vi "Facade.vi"(0 "Data In":T5, 2 "Display State In":T3={"X cursor"={"state"=enum."cursor and slider", "color"=0}, "Y cursor"={"state"=enum."cursor and slider", "color"=6618880}, "Scale Sliders"=FALSE}, 3 "Container State":T4) -> (6 "Data Out":T5, 7 "Display State Out":T3={"X cursor"={"state"=enum."cursor and slider", "color"=0}, "Y cursor"={"state"=enum."cursor and slider", "color"=6618880}, "Scale Sliders"=FALSE}, 8 "Action":T2)   [LabVIEW 2016, in "CursorImageControl.xctl"]
doc: "This is my documentation!!! Huzzahasdfasdf"
uses:
  CursorImageControl.xctl
  Data.ctl
  <vilib>/vision/Image Controls.llb/IMAQ Image.ctl
  <vilib>/_xctls/Container State.ctl
  State.ctl
  <vilib>/_xctls/Action.ctl
  <vilib>/Utility/miscctls.llb/LVPositionTypeDef.ctl
  PixelToMicron.vi
  <vilib>/_xctls/XControlSupport.lvlib
  <resource>/objmgr/IMAQImage.rc
panel:
  in  "X [mm]":dbl(slide) scale=-2.0..2.0 scale format="%#.2g"
  in  "Y [mm]":dbl(slide) scale=2.0..-2.0 scale format="%#.2g"
  out "Cursor Control":T1(plugin-control)
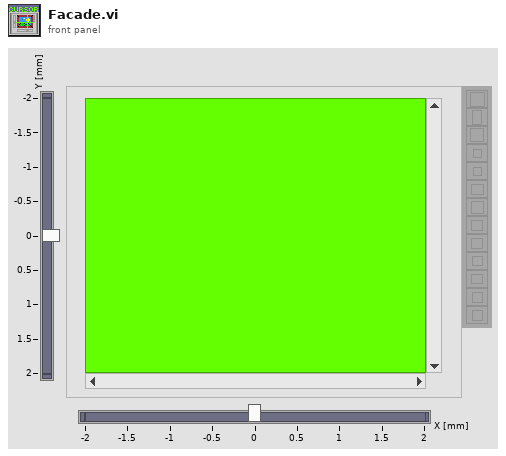
[diagram p1: front panel]
types:
  T1 = typedef "IMAQ Image.ctl" = refnum<image>
  T2 = typedef "XControlSupport.lvlib/Action.ctl" = cluster{"Data Changed?":bool, "State Changed?":bool, "Action Name":string}
  T3 = typedef "CursorImageControl.xctl/State.ctl" = cluster{"X cursor":cluster{"state":enum16{"cursor and slider", "cursor only", "hide all"}, "color":u32}, "Y cursor":cluster{"state":enum16{"cursor and slider", "cursor only", "hide all"}, "color":u32}, "Scale Sliders":bool}
  T4 = typedef "XControlSupport.lvlib/Container State.ctl" = cluster{"Indicator?":bool, "Run Mode?":bool, " Refnum":refnum<vi>}
  T5 = typedef "CursorImageControl.xctl/Data.ctl" = cluster{"Image":T1, "cursors":cluster{"X cursor":dbl, "Y cursor":dbl}}
  T6 = enum16{"cursor and slider", "cursor only", "hide all"}
  T7 = typedef "LVPositionTypeDef.ctl" = cluster{"Left":i32, "Top":i32}
  T8 = cluster{"state":enum16{"cursor and slider", "cursor only", "hide all"}, "state":enum16{"cursor and slider", "cursor only", "hide all"}}
  T9 = cluster{"Image":T1, cluster{"X [mm]":dbl, "Y [mm]":dbl}}
  T10 = typedef "LVBoundsTypeDef.ctl" = cluster{"Width":u32, "Height":u32}
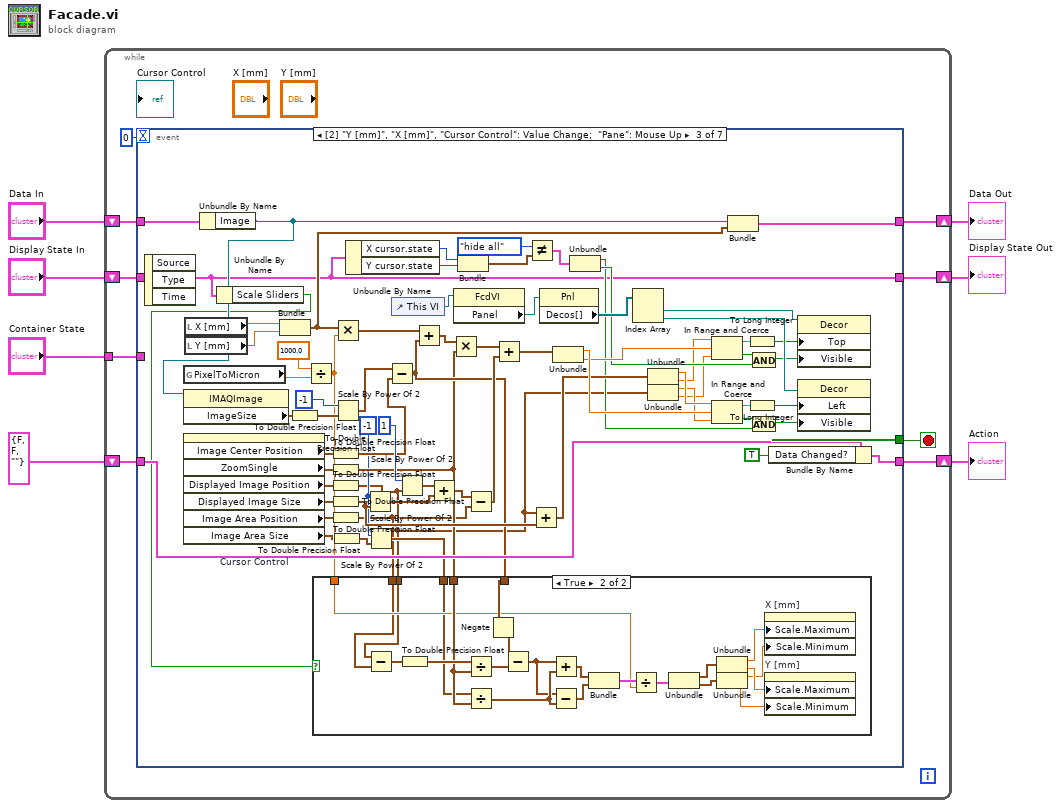
[diagram p0: block diagram]
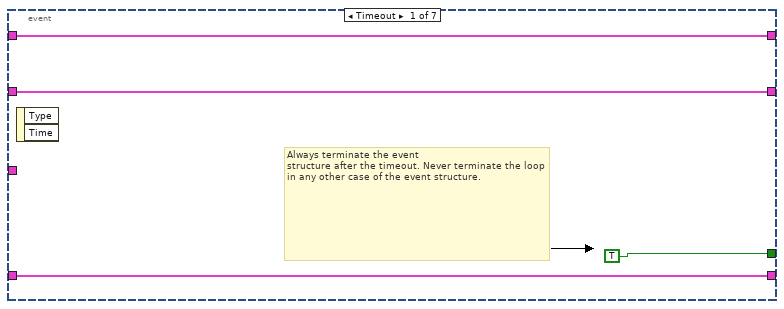
[diagram p2: hidden frame]
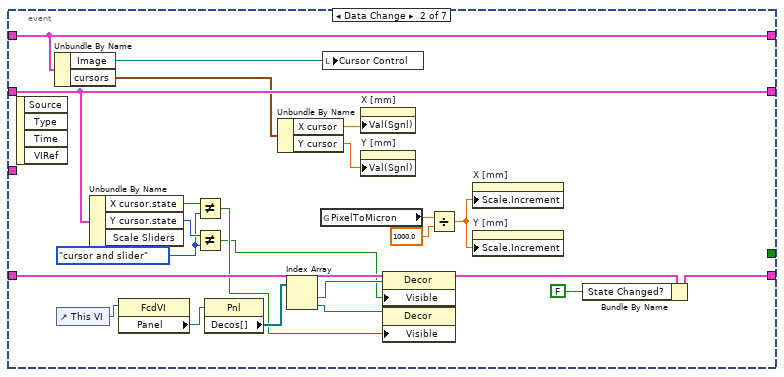
[diagram p3: hidden frame]
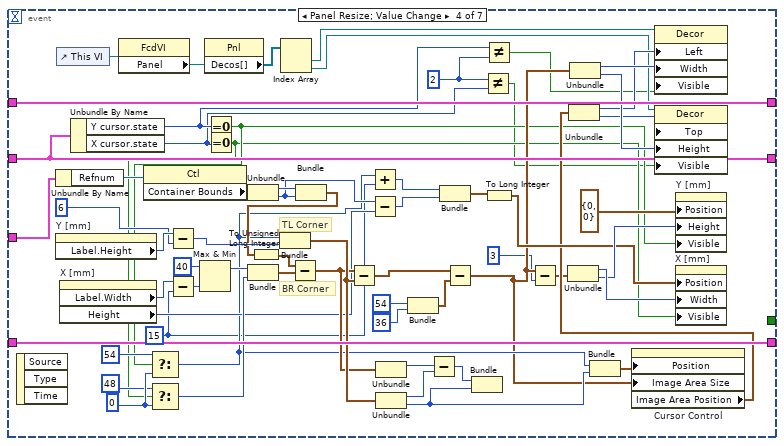
[diagram p5: hidden frame]
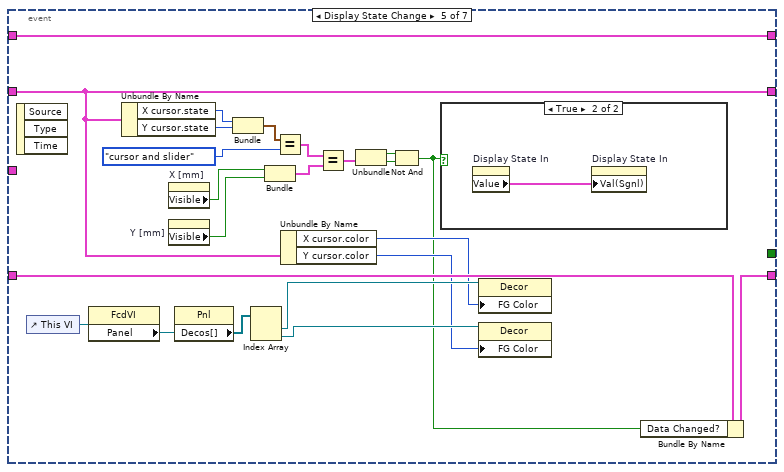
[diagram p6: hidden frame]
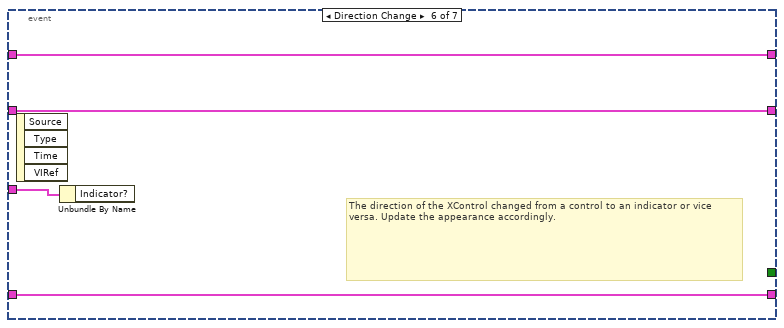
[diagram p8: hidden frame]
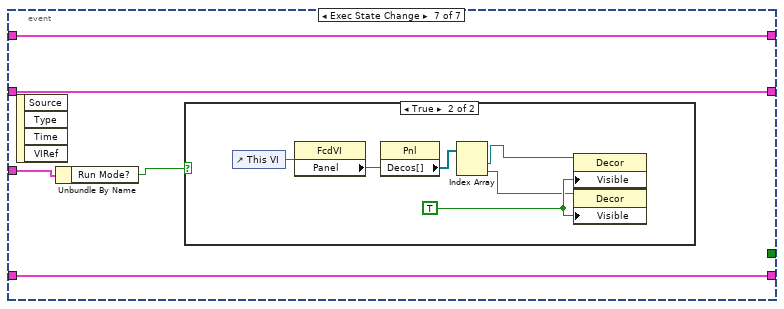
[diagram p9: hidden frame]
diagram:
  n1 = while {
    shift-right: [w15] -> w2
    shift-left: "Display State In" -> [w16]
    tunnel: "Container State" -> [w12]
    shift-right: [w8] -> w3
    shift-left: "Data In" -> [w9]
    shift-right: [w10] -> w1
    shift-left: T2 {"Data Changed?"=FALSE, "State Changed?"=FALSE, "Action Name"=""} ("Action") -> [w11]
    stop <- w14 stop-if-true
    n2 = event shown="[2] \"Y [mm]\", \"X [mm]\", \"Cursor Control\": Value Change;  \"Pane\": Mouse Up" {
      selector: _ -> [_ _ _ _ _ _ _]
      dyn-events: _ -> [_ _ _ _ _ _ _]
      timeout: 0 -> [_ _ _ _ _ _ _]
      tunnel: w16 -> [w18 w32 w56 w192 w201 w223 w226]
      tunnel: [w18 w32 w56 w192 w201 w223 w226] -> w15
      tunnel: [TRUE _ _ _ _ _ _] -> w14
      tunnel: w12 -> [_ _ _ w194 _ w224 w229]
      tunnel: w9 -> [w17 w39 w79 w196 w219 w221 w228]
      tunnel: [w17 w39 w62 w196 w219 w221 w228] -> w8
      tunnel: [w19 w41 w96 w195 w198 w222 w227] -> w10
      tunnel: w11 -> [w19 w42 w111 w195 w218 w222 w227]
      event Timeout {
        # "Always terminate the event\nstructure after the timeout. Never terminate the loop in any other case of the event structure."
        n3 = event-data() -> ()  [unwired: 1 in, 2 out]
      }
      event Data Change {
        w29 = T6."cursor and slider" ("X cursor.state")
        n4 = event-data() -> ()  [unwired: 1 in, 4 out]
        n5 = Unbundle By Name(w39) -> ("Image"=w26:T1, "cursors"=w21:cluster{"X cursor":dbl, "Y cursor":dbl})
        n6 = control-ref of="This VI"() -> (w34:refnum<vi>)
        n7 = Unbundle By Name(w32) -> ("X cursor.state"=w31:T6, "Y cursor.state"=w30:T6)  [unwired: 1 out]
        n8 = property class="FcdVI"(reference=w34) -> ("Panel"=w35:refnum<vi>)  [unwired: 1 in, 2 out]
        n9 = Not Equal?(x=w31, y=w29) -> (x != y?=w28:bool)
        n10 = Not Equal?(x=w30, y=w29) -> (x != y?=w27:bool)
        n11 = property class="Pnl"(reference=w35) -> ("Decos[]"=w36:refnum<vi>[])  [unwired: 1 in, 2 out]
        n12 = Unbundle By Name(w21) -> ("X cursor"=w22:dbl, "Y cursor"=w33:dbl)
        n13 = Index Array(array=w36) -> (element #1=w37:refnum<vi>, element #2=w38:refnum<vi>)  [unwired: 2 in]
        n14 = global read "PixelToMicron.vi" "PixelToMicron"() -> (w24:dbl)
        n15 = local write "Cursor Control"(w26) -> ()
        n16 = property on="X [mm]" class="Slide (strict)"("Val(Sgnl)"=w22) -> ()  [unwired: 2 in, 2 out]
        n17 = property on="Y [mm]" class="Slide (strict)"("Val(Sgnl)"=w33) -> ()  [unwired: 2 in, 2 out]
        n18 = property class="Decor"(reference=w37, "Visible"=w27) -> ()  [unwired: 1 in, 2 out]
        n19 = property class="Decor"(reference=w38, "Visible"=w28) -> ()  [unwired: 1 in, 2 out]
        n20 = Divide(x=w24, y=1000.0) -> (x/y=w23:dbl)
        n21 = property on="X [mm]" class="Slide (strict)"("Scale.Increment"=w23) -> ()  [unwired: 2 in, 2 out]
        n22 = property on="Y [mm]" class="Slide (strict)"("Scale.Increment"=w23) -> ()  [unwired: 2 in, 2 out]
        n23 = Bundle By Name(cluster=w42, "State Changed?"=FALSE) -> (w41:T2)
      }
      event "Y [mm]", "X [mm]", "Cursor Control": Value Change; Mouse Up {
        w47 = -1
        n24 = event-data() -> ()  [unwired: 1 in, 3 out]
        n25 = global read "PixelToMicron.vi" "PixelToMicron"() -> (w104:dbl)
        n26 = property on="Cursor Control" class="ImageControl"() -> ("Image Center Position"=w99:cluster{"X":u32, "Y":u32}, "ZoomSingle"=w100:cluster{"X":sgl, "Y":sgl}, "Displayed Image Position"=w92:cluster{"Left":i32, "Top":i32}, "Displayed Image Size"=w98:cluster{"Width":u32, "Height":u32}, "Image Area Position"=w90:cluster{"Left":i32, "Top":i32}, "Image Area Size"=w49:cluster{"Width":u32, "Height":u32})  [unwired: 2 in, 2 out]
        n27 = local read "X [mm]"() -> (w74:dbl)
        n28 = local read "Y [mm]"() -> (w73:dbl)
        n29 = Unbundle By Name(w79) -> ("Image"=w57:T1)
        n30 = property class="IMAQImage"(reference=w57) -> ("ImageSize"=w103:cluster{"x":i32, "y":i32})  [unwired: 1 in, 2 out]
        n31 = Unbundle By Name(w56) -> ("Scale Sliders"=w43:bool)
        n32 = Bundle("X [mm]"=w74, "Y [mm]"=w73) -> (w63:cluster{"X [mm]":dbl, "Y [mm]":dbl})  [unwired: 1 in]
        n33 = To Double Precision Float(number=w103) -> (double precision float=w101:cluster{"x":dbl, "y":dbl})
        n34 = Divide(x=1000.0, y=w104) -> (x/y=w50:dbl)
        n35 = To Double Precision Float(number=w99) -> (double precision float=w54:cluster{"X":dbl, "Y":dbl})
        n36 = To Double Precision Float(number=w100) -> (double precision float=w51:cluster{"X":dbl, "Y":dbl})
        n37 = To Double Precision Float(number=w92) -> (double precision float=w45:cluster{"Left":dbl, "Top":dbl})
        n38 = To Double Precision Float(number=w98) -> (double precision float=w80:cluster{"Width":dbl, "Height":dbl})
        n39 = To Double Precision Float(number=w90) -> (double precision float=w44:cluster{"Left":dbl, "Top":dbl})
        n40 = To Double Precision Float(number=w49) -> (double precision float=w48:cluster{"Width":dbl, "Height":dbl})
        n41 = Multiply(x=w63, y=w50) -> (x*y=w95:cluster{"X [mm]":dbl, "Y [mm]":dbl})
        n42 = Scale By Power Of 2(n=-1, x=w101) -> (x*2^n=w55:cluster{"x":dbl, "y":dbl})
        n43 = Unbundle By Name(w56) -> ("X cursor.state"=w71:T6, "Y cursor.state"=w72:T6)
        n44 = Scale By Power Of 2(n=w47, x=w80) -> (x*2^n=w89:cluster{"Width":dbl, "Height":dbl})
        n45 = Scale By Power Of 2(n=w47, x=w48) -> (x*2^n=w46:cluster{"Width":dbl, "Height":dbl})
        n46 = Subtract(x=w55, y=w54) -> (x-y=w52:cluster{dbl, dbl})
        n47 = case shown="True" w43 {
          tunnel: w52 -> [_ w118]
          tunnel: w51 -> [_ w117]
          tunnel: w50 -> [_ w116]
          tunnel: w46 -> [_ w115]
          tunnel: w45 -> [_ w114]
          tunnel: w44 -> [_ w113]
          frame False {
          }
          frame True {
            n48 = Subtract(x=w114, y=w113) -> (x-y=w128:cluster{"Left":dbl, "Top":dbl})
            n49 = To Double Precision Float(number=w128) -> (double precision float=w126:cluster{"Left":dbl, "Top":dbl})
            n50 = Divide(x=w126, y=w117) -> (x/y=w119:cluster{dbl, dbl})
            n51 = Divide(x=w115, y=w117) -> (x/y=w133:cluster{dbl, dbl})
            n52 = Negate(x=w118) -> (-x=w112:cluster{dbl, dbl})
            n53 = Subtract(x=w112, y=w119) -> (x-y=w120:cluster{dbl, dbl})
            n54 = Add(x=w120, y=w133) -> (x+y=w122:cluster{dbl, dbl})
            n55 = Subtract(x=w120, y=w133) -> (x-y=w121:cluster{dbl, dbl})
            n56 = Bundle(w122, w121) -> (w127:cluster{cluster{dbl, dbl}, cluster{dbl, dbl}})  [unwired: 1 in]
            n57 = Divide(x=w127, y=w116) -> (x/y=w123:cluster{cluster{dbl, dbl}, cluster{dbl, dbl}})
            n58 = Unbundle(w123) -> (w125:cluster{dbl, dbl}, w124:cluster{dbl, dbl})
            n59 = Unbundle(w125) -> (w132:dbl, w131:dbl)
            n60 = Unbundle(w124) -> (w130:dbl, w129:dbl)
            n61 = property on="X [mm]" class="Slide (strict)"("Scale.Maximum"=w132, "Scale.Minimum"=w130) -> ()  [unwired: 2 in, 2 out]
            n62 = property on="Y [mm]" class="Slide (strict)"("Scale.Maximum"=w131, "Scale.Minimum"=w129) -> ()  [unwired: 2 in, 2 out]
          }
        }
        n63 = control-ref of="This VI"() -> (w110:refnum<vi>)
        n64 = Scale By Power Of 2(n=1, x=w45) -> (x*2^n=w83:cluster{"Left":dbl, "Top":dbl})
        n65 = Add(x=w95, y=w52) -> (x+y=w53:cluster{dbl, dbl})
        n66 = Add(x=w83, y=w89) -> (x+y=w81:cluster{dbl, dbl})
        n67 = Multiply(x=w53, y=w51) -> (x*y=w97:cluster{dbl, dbl})
        n68 = property class="FcdVI"(reference=w110) -> ("Panel"=w109:refnum<vi>)  [unwired: 1 in, 2 out]
        n69 = Bundle("state"=w71, "state"=w72) -> (w69:T8)  [unwired: 1 in]
        n70 = Subtract(x=w81, y=w44) -> (x-y=w84:cluster{dbl, dbl})
        n71 = Add(x=w97, y=w84) -> (x+y=w91:cluster{dbl, dbl})
        n72 = Not Equal?(x=T6."hide all" ("X cursor.state"), y=w69) -> (x != y?=w66:cluster{"state":bool, "state":bool})
        n73 = Add(x=w45, y=w80) -> (x+y=w75:cluster{dbl, dbl})
        n74 = property class="Pnl"(reference=w109) -> ("Decos[]"=w108:refnum<vi>[])  [unwired: 1 in, 2 out]
        n75 = Unbundle(w91) -> (w88:dbl, w87:dbl)
        n76 = Unbundle(w66) -> ("state"=w64:bool, "state"=w65:bool)
        n77 = Index Array(array=w108) -> (element #1=w107:refnum<vi>, element #2=w106:refnum<vi>)  [unwired: 2 in]
        n78 = Unbundle(w75) -> (w61:dbl, w59:dbl)
        n79 = Unbundle(w45) -> ("Left"=w60:dbl, "Top"=w58:dbl)
        n80 = In Range and Coerce(upper limit=w59, x=w87, lower limit=w58) -> (coerced(x)=w86:dbl, In Range?=w76:bool)
        n81 = In Range and Coerce(upper limit=w61, x=w88, lower limit=w60) -> (coerced(x)=w85:dbl, In Range?=w77:bool)
        n82 = Bundle("Image"=w57, w63) -> (w62:T9)  [unwired: 1 in]
        n83 = To Long Integer(number=w86) -> (32bit integer=w94:i32)
        n84 = To Long Integer(number=w85) -> (32bit integer=w93:i32)
        n85 = And(x=w76, y=w65) -> (x .and. y?=w68:bool)
        n86 = And(x=w77, y=w64) -> (x .and. y?=w67:bool)
        n87 = Bundle By Name(cluster=w111, "Data Changed?"=TRUE) -> (w96:T2)
        n88 = property class="Decor"(reference=w107, "Top"=w94, "Visible"=w68) -> ()  [unwired: 1 in, 2 out]
        n89 = property class="Decor"(reference=w106, "Left"=w93, "Visible"=w67) -> ()  [unwired: 1 in, 2 out]
      }
      event Panel Resize; Value Change {
        w136 = u16 2
        w156 = u32 15 ("y")
        w191 = u32 0
        # "BR Corner"
        # "TL Corner"
        n90 = event-data() -> ()  [unwired: 1 in, 3 out]
        n91 = Unbundle By Name(w194) -> ("Refnum"=w193:refnum<vi>)
        n92 = property on="Y [mm]" class="Slide (strict)"() -> ("Label.Height"=w189:u32)  [unwired: 2 in, 2 out]
        n93 = control-ref of="This VI"() -> (w151:refnum<vi>)
        n94 = property on="X [mm]" class="Slide (strict)"() -> ("Label.Width"=w188:u32, "Height"=w166:u32)  [unwired: 2 in, 2 out]
        n95 = Unbundle By Name(w192) -> ("Y cursor.state"=w138:T6, "X cursor.state"=w137:T6)
        n96 = property class="FcdVI"(reference=w151) -> ("Panel"=w152:refnum<vi>)  [unwired: 1 in, 2 out]
        n97 = property class="Ctl"(reference=w193) -> ("Container Bounds"=w181:T10)  [unwired: 1 in, 2 out]
        n98 = Subtract(x=w189, y=u32 6) -> (x-y=w184:u32)
        n99 = Subtract(x=w188, y=w156) -> (x-y=w186:u32)
        n100 = Max & Min(x=u32 40, y=w186) -> (max(x,y)=w183:u32)  [unwired: 1 out]
        n101 = property class="Pnl"(reference=w152) -> ("Decos[]"=w153:refnum<vi>[])  [unwired: 1 in, 2 out]
        n102 = Equal To 0?(x=w138) -> (x = 0?=w140:bool)
        n103 = Select(t=u32 54, s=w140, f=w191) -> (s? t:f=w162:u32)
        n104 = Equal To 0?(x=w137) -> (x = 0?=w139:bool)
        n105 = Select(t=u32 48, s=w139, f=w191) -> (s? t:f=w182:u32)
        n106 = Unbundle(w181) -> ("Width"=w180:u32, "Height"=w167:u32)
        n107 = Bundle(w183, w182) -> (w175:cluster{u32, u32})  [unwired: 1 in]
        n108 = Bundle(w162, w184) -> (w173:cluster{u32, u32})  [unwired: 1 in]
        n109 = Index Array(array=w153) -> (element #1=w142:refnum<vi>, element #2=w141:refnum<vi>)  [unwired: 2 in]
        n110 = Bundle("Width"=w180, "Height"=w167) -> (w179:cluster{"Width":u32, "Height":u32})  [unwired: 1 in]
        n111 = To Unsigned Long Integer(number=w179) -> (unsigned 32bit integer=w174:cluster{"Width":u32, "Height":u32})
        n112 = Subtract(x=w174, y=w175) -> (x-y=w172:cluster{u32, u32})
        n113 = Subtract(x=w172, y=w173) -> (x-y=w178:cluster{u32, u32})
        n114 = Add(x=w162, y=w156) -> (x+y=w161:u32)
        n115 = Subtract(x=w167, y=w166) -> (x-y=w160:u32)
        n116 = Unbundle(w172) -> (w171:u32)  [unwired: 1 out]
        n117 = Unbundle(w173) -> (w170:u32, w155:u32)
        n118 = Bundle(u32 54, u32 36) -> (w157:cluster{u32, u32})  [unwired: 1 in]
        n119 = Subtract(x=w171, y=w170) -> (x-y=w169:u32)
        n120 = Bundle(w161, w160) -> (w165:cluster{u32, u32})  [unwired: 1 in]
        n121 = Subtract(x=w178, y=w157) -> (x-y=w144:cluster{u32, u32})
        n122 = Bundle(w169, w155) -> ()  [unwired: 1 in, 1 out]
        n123 = Not Equal?(x=w136, y=w137) -> (x != y?=w134:bool)
        n124 = Not Equal?(x=w138, y=w136) -> (x != y?=w135:bool)
        n125 = To Long Integer(number=w165) -> (32bit integer=w164:cluster{i32, i32})
        n126 = Subtract(x=w144, y=u32 3) -> (x-y=w145:cluster{u32, u32})
        n127 = Unbundle(w145) -> (w177:u32, w176:u32)
        n128 = Unbundle(w144) -> (w150:u32, w149:u32)
        n129 = Bundle(w162, w155) -> (w163:cluster{u32, u32})  [unwired: 1 in]
        n130 = property on="Cursor Control" class="ImageControl"("Position"=w163, "Image Area Size"=w144) -> ("Image Area Position"=w146:cluster{"Left":i32, "Top":i32})  [unwired: 2 in, 2 out]
        n131 = Unbundle(w146) -> ("Left"=w148:i32, "Top"=w147:i32)
        n132 = property class="Decor"(reference=w142, "Left"=w148, "Width"=w150, "Visible"=w135) -> ()  [unwired: 1 in, 2 out]
        n133 = property class="Decor"(reference=w141, "Top"=w147, "Height"=w149, "Visible"=w134) -> ()  [unwired: 1 in, 2 out]
        n134 = property on="Y [mm]" class="Slide (strict)"("Position"=T7 {"Left"=0, "Top"=0}, "Height"=w176, "Visible"=w140) -> ()  [unwired: 2 in, 2 out]
        n135 = property on="X [mm]" class="Slide (strict)"("Position"=w164, "Width"=w177, "Visible"=w139) -> ()  [unwired: 2 in, 2 out]
      }
      event Display State Change {
        n136 = event-data() -> ()  [unwired: 1 in, 3 out]
        n137 = control-ref of="This VI"() -> (w215:refnum<vi>)
        n138 = property class="FcdVI"(reference=w215) -> ("Panel"=w216:refnum<vi>)  [unwired: 1 in, 2 out]
        n139 = Unbundle By Name(w201) -> ("X cursor.state"=w211:T6, "Y cursor.state"=w212:T6)
        n140 = property on="X [mm]" class="Slide (strict)"() -> ("Visible"=w209:bool)  [unwired: 2 in, 2 out]
        n141 = property on="Y [mm]" class="Slide (strict)"() -> ("Visible"=w208:bool)  [unwired: 2 in, 2 out]
        n142 = property class="Pnl"(reference=w216) -> ("Decos[]"=w217:refnum<vi>[])  [unwired: 1 in, 2 out]
        n143 = Bundle("state"=w211, "state"=w212) -> (w202:T8)  [unwired: 1 in]
        n144 = Index Array(array=w217) -> (element #1=w214:refnum<vi>, element #2=w213:refnum<vi>)  [unwired: 2 in]
        n145 = Bundle("Visible"=w209, "Visible"=w208) -> (w206:cluster{"Visible":bool, "Visible":bool})  [unwired: 1 in]
        n146 = Equal?(x=w202, y=T6."cursor and slider" ("Y cursor.state")) -> (x = y?=w207:cluster{"state":bool, "state":bool})
        n147 = Unbundle By Name(w201) -> ("X cursor.color"=w200:u32, "Y cursor.color"=w199:u32)
        n148 = Equal?(x=w207, y=w206) -> (x = y?=w205:cluster{bool, bool})
        n149 = Unbundle(w205) -> (w204:bool, w203:bool)
        n150 = Not And(1:w203, 2:w204) -> (0:w197:bool)
        n151 = case shown="True" w197 {
          frame False {
          }
          frame True {
            n152 = property on="Display State In" class="Clust (strict)"() -> ("Value"=w220:T3)  [unwired: 2 in, 2 out]
            n153 = property on="Display State In" class="Clust (strict)"("Val(Sgnl)"=w220) -> ()  [unwired: 2 in, 2 out]
          }
        }
        n154 = property class="Decor"(reference=w214, "FG Color"=w200) -> ()  [unwired: 1 in, 2 out]
        n155 = property class="Decor"(reference=w213, "FG Color"=w199) -> ()  [unwired: 1 in, 2 out]
        n156 = Bundle By Name(cluster=w218, "Data Changed?"=w197) -> (w198:T2)
      }
      event Direction Change {
        # "The direction of the XControl changed from a control to an indicator or vice versa. Update the appearance accordingly."
        n157 = event-data() -> ()  [unwired: 1 in, 4 out]
        n158 = Unbundle By Name(w224) -> ()  [unwired: 1 out]
      }
      event Exec State Change {
        n159 = event-data() -> ()  [unwired: 1 in, 4 out]
        n160 = Unbundle By Name(w229) -> ("Run Mode?"=w225:bool)
        n161 = case shown="True" w225 {
          frame False {
          }
          frame True {
            w235 = TRUE
            n162 = control-ref of="This VI"() -> (w232:refnum<vi>)
            n163 = property class="FcdVI"(reference=w232) -> ("Panel"=w233:refnum<vi>)  [unwired: 1 in, 2 out]
            n164 = property class="Pnl"(reference=w233) -> ("Decos[]"=w234:refnum<vi>[])  [unwired: 1 in, 2 out]
            n165 = Index Array(array=w234) -> (element #1=w231:refnum<vi>, element #2=w230:refnum<vi>)  [unwired: 2 in]
            n166 = property class="Decor"(reference=w231, "Visible"=w235) -> ()  [unwired: 1 in, 2 out]
            n167 = property class="Decor"(reference=w230, "Visible"=w235) -> ()  [unwired: 1 in, 2 out]
          }
        }
      }
    }
  }
  "Display State Out" <- w2
  "Data Out" <- w3
  "Action" <- w1
